vi "cancel.vi"(8 "error in":errorcluster, 11 "null task token in":refnum<class "null task token.lvclass">) -> (0 "error out":errorcluster, 3 "null task token out":refnum<class "null task token.lvclass">)   [LabVIEW 2013, in "null task token.lvclass"]
uses:
  null task token.lvclass
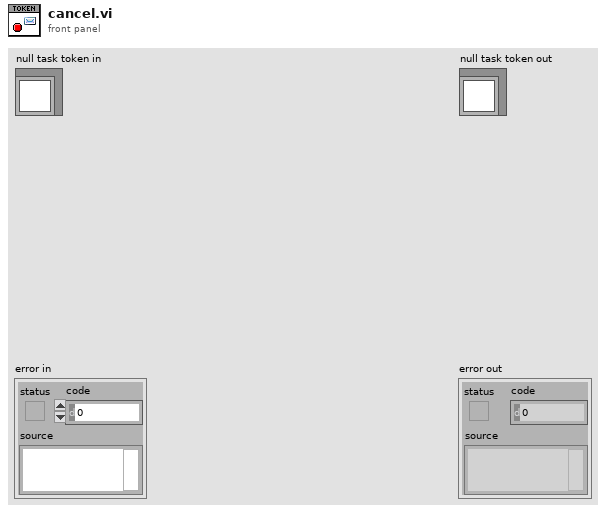
[diagram p1: front panel]
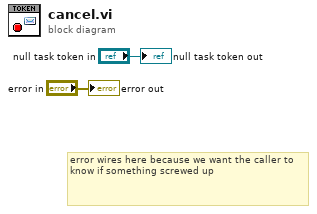
[diagram p0: block diagram]
diagram:
  # "error wires here because we want the caller to know if something screwed up"
  "error out" <- "error in"
  "null task token out" <- "null task token in"
